vi "DownsampleStage2_5160_singlechannel_old.vi"(8 "valid in":bool, 9 "reset":bool, 11 "Element":fxp<+/-,20,16>[](array[numeric])=[0.0, 0.0, 0.0, 0.0]) -> (0 "valid out":bool, 3 "Element 1":u64)   [LabVIEW 2013]
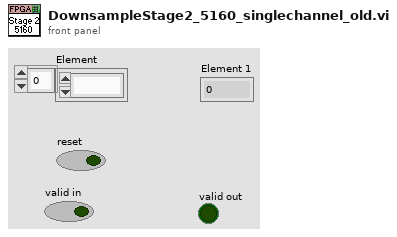
[diagram p1: front panel]
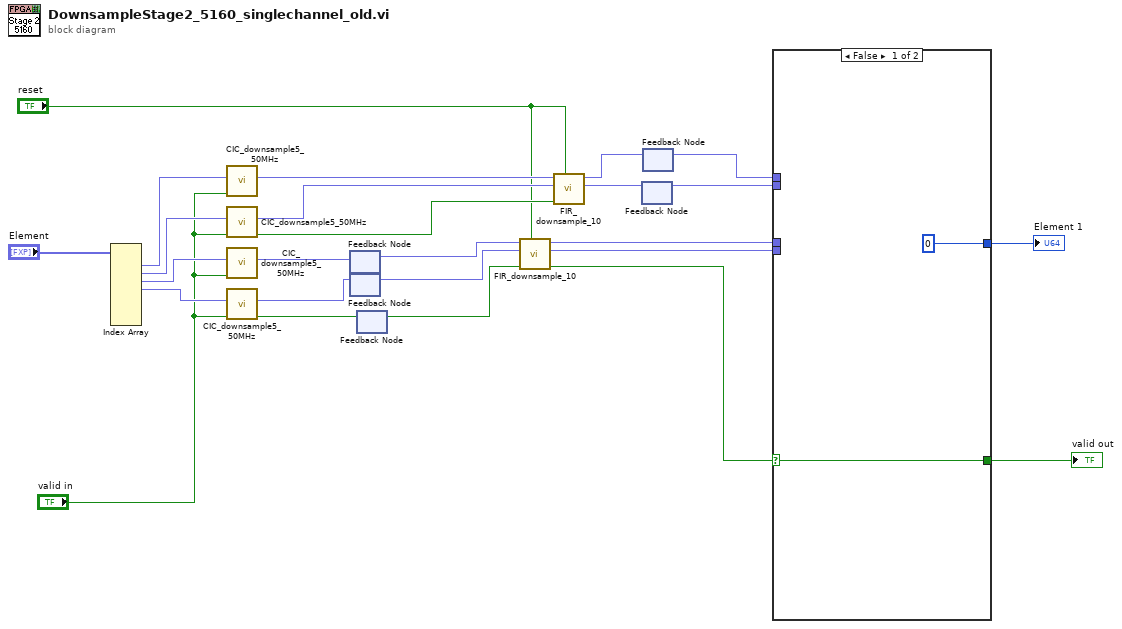
[diagram p0: block diagram]
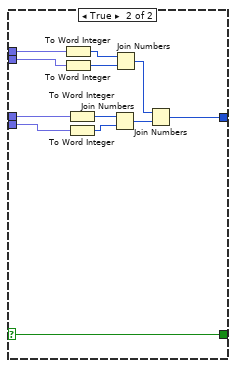
[diagram p2: hidden frame]
diagram:
  n1 = Index Array(array="Element") -> (element #1=w22:fxp<+/-,20,16>, element #2=w21:fxp<+/-,20,16>, element #3=w20:fxp<+/-,20,16>, element #4=w19:fxp<+/-,20,16>)  [unwired: 8 in, 4 out]
  n2 = call "CIC_downsample5_50MHz.vi"("valid in"="valid in", "din"=w22) -> ("dout"=w17:fxp<+/-,25,19>)  [unwired: 7 in, 2 out]
  n3 = call "CIC_downsample5_50MHz.vi"("valid in"="valid in", "din"=w21) -> ("valid out"=w15:bool, "dout"=w16:fxp<+/-,25,19>)  [unwired: 7 in, 1 out]
  n4 = call "CIC_downsample5_50MHz.vi"("valid in"="valid in", "din"=w20) -> ("dout"=w5:fxp<+/-,25,19>)  [unwired: 7 in, 2 out]
  n5 = call "CIC_downsample5_50MHz.vi"("valid in"="valid in", "din"=w19) -> ("valid out"=w9:bool, "dout"=w7:fxp<+/-,25,19>)  [unwired: 7 in, 1 out]
  n6 = feedback #1() -> (w4:fxp<+/-,25,19>)  [unwired: 1 in]
  n7 = feedback-in #1(w5) -> ()
  n8 = feedback #2() -> (w6:fxp<+/-,25,19>)  [unwired: 1 in]
  n9 = feedback-in #2(w7) -> ()
  n10 = feedback #3() -> (w8:bool)  [unwired: 1 in]
  n11 = feedback-in #3(w9) -> ()
  n12 = call "FIR_downsample_10.vi"("reset"="reset", "valid in"=w8, "Q in"=w6, "I in"=w4) -> ("valid out"=w1:bool, "Q out"=w2:fxp<+/-,16,16>, "I out"=w3:fxp<+/-,16,16>)  [unwired: 4 in, 1 out]
  n13 = call "FIR_downsample_10.vi"("reset"="reset", "valid in"=w15, "Q in"=w16, "I in"=w17) -> ("Q out"=w12:fxp<+/-,16,16>, "I out"=w13:fxp<+/-,16,16>)  [unwired: 4 in, 2 out]
  n14 = feedback #4() -> (w10:fxp<+/-,16,16>)  [unwired: 1 in]
  n15 = feedback-in #4(w12) -> ()
  n16 = feedback-in #5(w13) -> ()
  n17 = feedback #5() -> (w11:fxp<+/-,16,16>)  [unwired: 1 in]
  n18 = case shown="False" w1 {
    selector: w1 -> [w27 w28]
    tunnel: w11 -> [_ w33]
    tunnel: w10 -> [_ w32]
    tunnel: w3 -> [_ w31]
    tunnel: w2 -> [_ w30]
    tunnel: [u64 0 w29] -> w24
    tunnel: [w27 w28] -> w23
    frame False {
    }
    frame True {
      n19 = To Word Integer(number=w33) -> (16bit integer=w38:i16)
      n20 = To Word Integer(number=w32) -> (16bit integer=w39:i16)
      n21 = To Word Integer(number=w31) -> (16bit integer=w37:i16)
      n22 = To Word Integer(number=w30) -> (16bit integer=w36:i16)
      n23 = Join Numbers(hi=w37, lo=w36) -> ((hi.lo)=w34:u32)
      n24 = Join Numbers(hi=w38, lo=w39) -> ((hi.lo)=w35:u32)
      n25 = Join Numbers(hi=w35, lo=w34) -> ((hi.lo)=w29:u64)
    }
  }
  "Element 1" <- w24
  "valid out" <- w23
